vi "SR Flip Flop.vi"(9 "Enable":bool, 10 "Reset":bool, 11 "Set":bool) -> (3 "Output":bool)   [LabVIEW 2014, in "memLib.lvlib"]
uses:
  memLib.lvlib
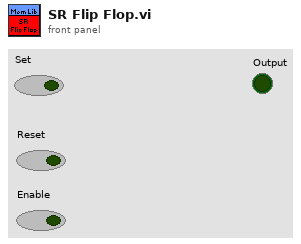
[diagram p1: front panel]
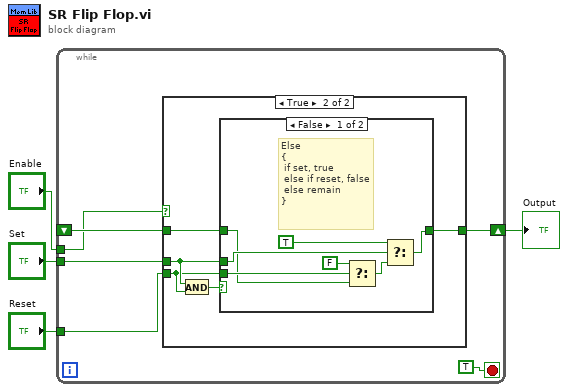
[diagram p0: block diagram]
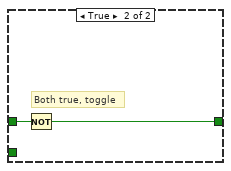
[diagram p3: hidden frame]
diagram:
  n1 = while {
    tunnel: "Set" -> [w9]
    shift-right: [w5] -> w1
    shift-left: _ -> [w7]
    tunnel: "Reset" -> [w8]
    tunnel: "Enable" -> [w6]
    stop <- TRUE stop-if-true
    n2 = case shown="True" w6 {
      tunnel: w9 -> [_ w13]
      tunnel: w8 -> [_ w12]
      tunnel: w7 -> [w11 w15]
      tunnel: [w11 w14] -> w5
      frame False {
        # "if not enabled, no change."
      }
      frame True {
        n3 = And(x=w13, y=w12) -> (x .and. y?=w16:bool)
        n4 = case shown="False" w16 {
          tunnel: w15 -> [w18 w25]
          tunnel: [w17 w24] -> w14
          tunnel: w13 -> [w22 _]
          tunnel: w12 -> [w19 _]
          frame False {
            # "Else\n{\n if set, true\n else if reset, false\n else remain\n}"
            n5 = Select(t=FALSE, s=w19, f=w18) -> (s? t:f=w23:bool)
            n6 = Select(t=TRUE, s=w22, f=w23) -> (s? t:f=w17:bool)
          }
          frame True {
            # "Both true, toggle"
            n7 = Not(x=w25) -> (.not. x?=w24:bool)
          }
        }
      }
    }
  }
  "Output" <- w1
